vi "Add Header Write.vi"(8 "error in":errorcluster, 10 "Api Token":string="8y3UfvlU-s_u9u_oxA6shSxOW3EspqNUnOF1NvG3HuRk3uhql6GwvIuXxEX0eFPkzaJQUr8iPPkS1eW6XzXgRw==", 11 "client handle in":T1) -> (0 "error out":errorcluster, 3 "client handle out":T1)   [LabVIEW 2020, in "InfluxDB v2 Client.lvlib"]
doc: "Creates the header for query"
uses:
  InfluxDB v2 Client.lvlib
  <vilib>/httpClient/ClientHandle.ctl
  <vilib>/httpClient/LabVIEWHTTPClient.lvlib
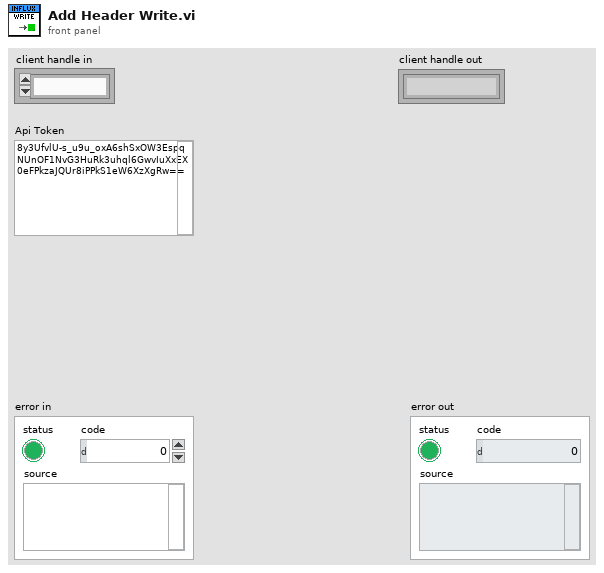
[diagram p1: front panel]
types:
  T1 = typedef "LabVIEWHTTPClient.lvlib/ClientHandle.ctl" = refnum<k1>
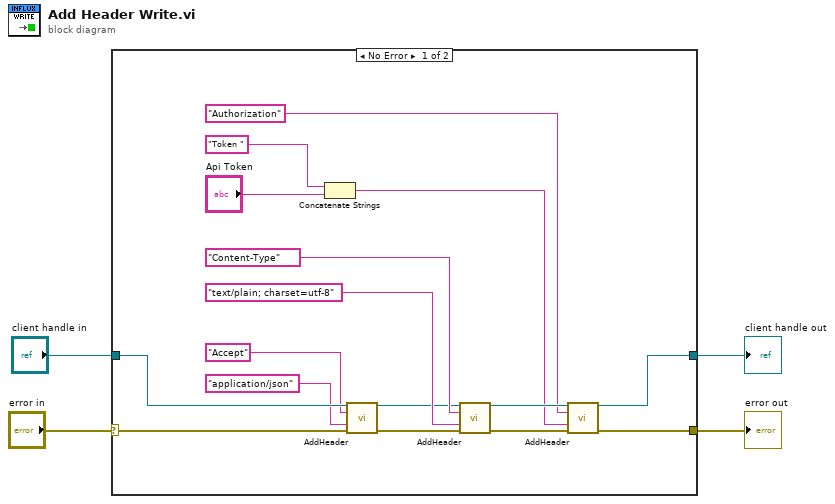
[diagram p0: block diagram]
diagram:
  n1 = case shown="No Error" "error in" {
    selector: "error in" -> [w9 w21]
    tunnel: [w13 w21] -> w3
    tunnel: "client handle in" -> [w8 w22]
    tunnel: [w11 w22] -> w1
    frame No Error {
      n2 = Concatenate Strings("Token ", "Api Token") -> (w14:string)
      n3 = call <vilib>:"AddHeader.vi"("client handle"=w8, "header"="Accept" ("value"), "value"="application/json", "error in (no error)"=w9) -> ("client handle out"=w5:T1, "error out"=w10:errorcluster)  [unwired: 10 in]
      n4 = call <vilib>:"AddHeader.vi"("client handle"=w5, "header"="Content-Type", "value"="text/plain; charset=utf-8", "error in (no error)"=w10) -> ("client handle out"=w18:T1, "error out"=w17:errorcluster)  [unwired: 10 in]
      n5 = call <vilib>:"AddHeader.vi"("client handle"=w18, "header"="Authorization", "value"=w14, "error in (no error)"=w17) -> ("client handle out"=w11:T1, "error out"=w13:errorcluster)  [unwired: 10 in]
    }
    frame Error {
    }
  }
  "client handle out" <- w1
  "error out" <- w3
